vi "Convert CSV to dynamic data type iso.vi"(1 "Input Datafile Separator":enum32{"CSV", "TSV"}(radio), 2 "column containing\nforce data":i32=1, 3 "selected path":path) -> (0 "Dynamic Data Type":dynamicdata(waveform))   [LabVIEW 2016]
uses:
  <vilib>/Utility/file.llb/Read Delimited Spreadsheet (string).vi
  <vilib>/Utility/file.llb/Read Delimited Spreadsheet (DBL).vi
panel:
  out "x-y":dbl
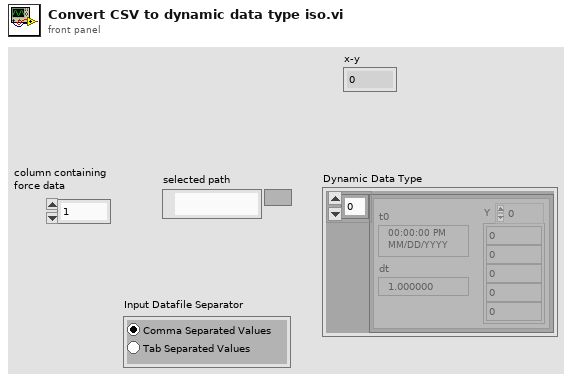
[diagram p1: front panel]
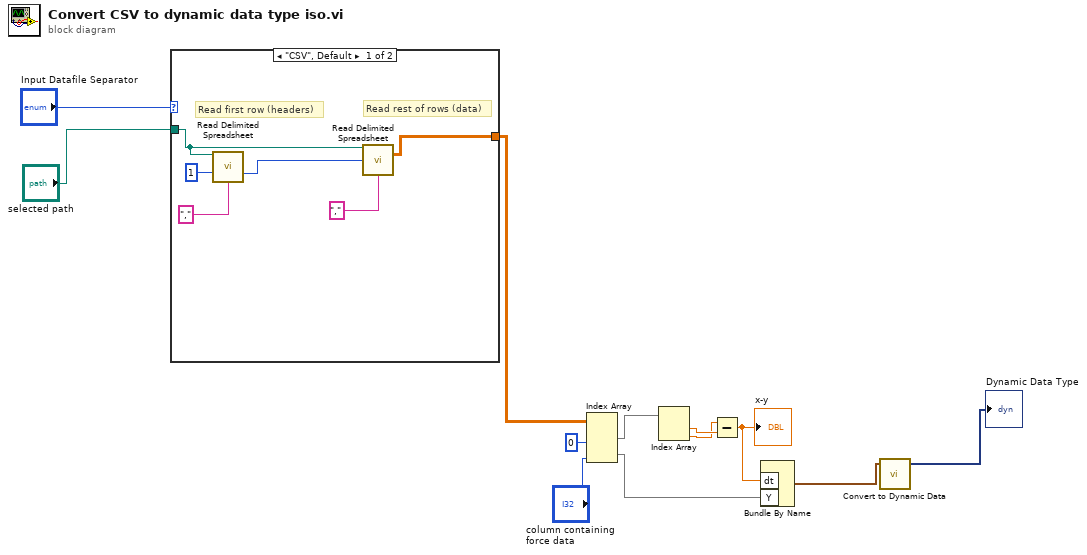
[diagram p0: block diagram]
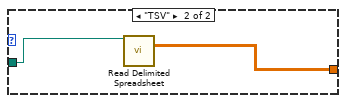
[diagram p2: hidden frame]
diagram:
  n1 = case shown="\"CSV\", Default" "Input Datafile Separator" {
    tunnel: "selected path" -> [w16 w20]
    tunnel: [w17 w19] -> w10
    frame "CSV", Default {
      # "Read rest of rows (data)"
      # "Read first row (headers)"
      n2 = call-poly <vilib>:"Read Delimited Spreadsheet.vi"("file path (dialog if empty)"=w16, "number of rows (all:-1)"=1, "delimiter (\\t)"="," ("delimiter (\\t)")) -> ("mark after read (chars.)"=w14:i32)  [unwired: 7 in, 5 out]
      n3 = call-poly <vilib>:"Read Delimited Spreadsheet.vi"("file path (dialog if empty)"=w16, "start of read offset (chars.:0)"=w14, "delimiter (\\t)"="," ("delimiter")) -> ("all rows"=w17:dbl[][])  [unwired: 7 in, 5 out]
    }
    frame "TSV" {
      n4 = call-poly <vilib>:"Read Delimited Spreadsheet.vi"("file path (dialog if empty)"=w20) -> ("all rows"=w19:dbl[][])  [unwired: 9 in, 5 out]
    }
  }
  n5 = Index Array(array=w10, index (col) #1=0 ("disabled index (col)"), index (col) #2="column containing\nforce data") -> (element #1=w9:dbl[], element #2=w5:dbl[])  [unwired: 2 in]
  n6 = Index Array(array=w9) -> (element #1=w8:dbl, element #2=w7:dbl)  [unwired: 2 in]
  n7 = Subtract(x=w7, y=w8) -> (x-y=w6:dbl)
  "x-y" <- w6
  n8 = Bundle By Name("dt"=w6, "Y"=w5) -> (w1:waveform(dbl))  [unwired: 1 in]
  n9 = call "Convert to Dynamic Data"("Waveform"=w1) -> ("Dynamic Data Type"=→"Dynamic Data Type":dynamicdata)  [unwired: 3 in]
